vi "ConvertVItoHTML.vi"(0 "vi name":string) -> (1 "Htm log name":string, 2 "Server Name":string)   [LabVIEW 2012]
doc: "Converts VI name to an HTML name and a server name"
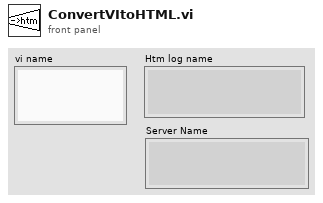
[diagram p1: front panel]
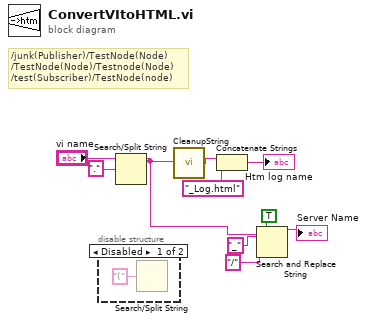
[diagram p0: block diagram]
diagram:
  # "/junk(Publisher)/TestNode(Node)\n/TestNode(Node)/Testnode(Node)\n/test(Subscriber)/TestNode(node)"
  n1 = disable-structure shown="Disabled" {
    frame Disabled {
      n2 = Search/Split String(search string/char (-)="(") -> ()  [unwired: 2 in, 3 out]
    }
    frame Enabled {
    }
  }
  n3 = Search/Split String(string="vi name", search string/char (-)=".") -> (substring before match=w3:string)  [unwired: 1 in, 2 out]
  n4 = call "CleanupString.vi"("String"=w3) -> ("url"=w2:string)
  n5 = Concatenate Strings(w2, "_Log.html" ("string")) -> (→"Htm log name":string)
  n6 = Search and Replace String(replace all?=TRUE ("replace all? (F)"), input string=w3, search string="_", replace string="/" ("replace string (\"\")")) -> (result string=→"Server Name":string)  [unwired: 4 in, 3 out]
